vi "hex string to num.vi"(8 "error in (no error)":errorcluster caption="에러 입력(에러 없음)", 9 "min byte (1)":u8=1, 10 "max byte (1)":u8=1, 11 "string":string) -> (0 "error out":errorcluster caption="에러 출력", 1 "byte":u8, 2 "error":bool, 3 "num":u32)   [LabVIEW 2020, in "Script Line.lvclass"]
uses:
  Script Line.lvclass
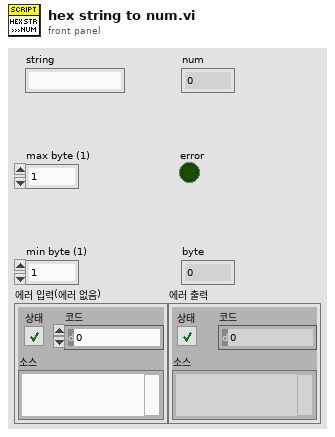
[diagram p1: front panel]
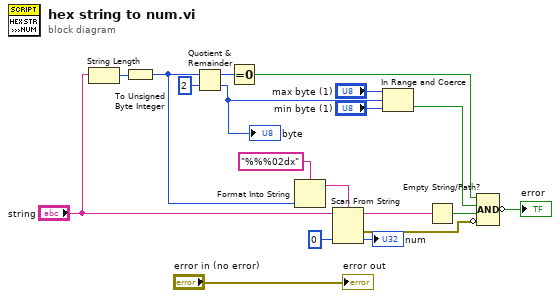
[diagram p0: block diagram]
diagram:
  n1 = String Length(string="string") -> (length=w7:i32)
  n2 = To Unsigned Byte Integer(number=w7) -> (unsigned 8bit integer=w2:u8)
  n3 = Quotient & Remainder(x=w2, y=u8 2) -> (x-y*floor(x/y)=w11:u8, floor(x/y)=w6:u8)
  "byte" <- w6
  n4 = Equal To 0?(x=w11) -> (x = 0?=w10:bool)
  n5 = Format Into String(format string="%%%02dx" ("포맷 문자열"), w2) -> (resulting string=w8:string)  [unwired: 2 in, 1 out]
  n6 = Scan From String(format string=w8, input string="string", default 1=u32 0) -> (remaining string=w18:string, error out=w16:errorcluster, output 1=→"num":u32)  [unwired: 2 in, 1 out]
  n7 = In Range and Coerce(upper limit="max byte (1)", x=w6, lower limit="min byte (1)") -> (In Range?=w5:bool)  [unwired: 1 out]
  n8 = Empty String/Path?(string/path=w18) -> (empty?=w17:bool)
  n9 = Compound Arithmetic op=AND(w10, w5, w17, invert w16) -> (invert →"error":bool)
  "error out" <- "error in (no error)"
